vi "FPGA Settings.vi"(8 "error in":errorcluster, 9 "Action":T2, 10 "FPGA Settings":T1={"Bitfile path"=path "", "RIO Device Address"="RIO0", "Group"=FALSE}, 11 "VS Engine in":refnum<class "VS Engine.lvclass">) -> (0 "error out":errorcluster, 2 "FPGA Settings":T1, 3 "VS Engine out":refnum<class "VS Engine.lvclass">)   [LabVIEW 2024, in "VS Engine Abstraction.lvlib" / "VS Engine.lvclass"]
uses:
  VS Engine.lvclass
  VS Engine.lvclass/VS Engine.ctl
  <vilib>/NI VeriStand/Custom Device API/Custom Device API.lvlib
  Addon Shared/SubVIs/Constants.vi
  Addon Shared/FPGA Addon Shared.lvlib
  <vilib>/NI VeriStand/Custom Device API/Set Item Property (Boolean).vi
  <vilib>/NI VeriStand/Custom Device API/Get Item Property (Boolean).vi
  <vilib>/NI VeriStand/Custom Device API/Get Item Property (String).vi
  <vilib>/NI VeriStand/Custom Device API/Set Item Property (String).vi
  <vilib>/NI VeriStand/Custom Device API/Set Item Property (Path).vi
  <vilib>/NI VeriStand/Custom Device API/Get Item Property (Path).vi
  Addon Shared/Types/FPGA Settings.ctl
  Addon Shared/Types/FG Action.ctl
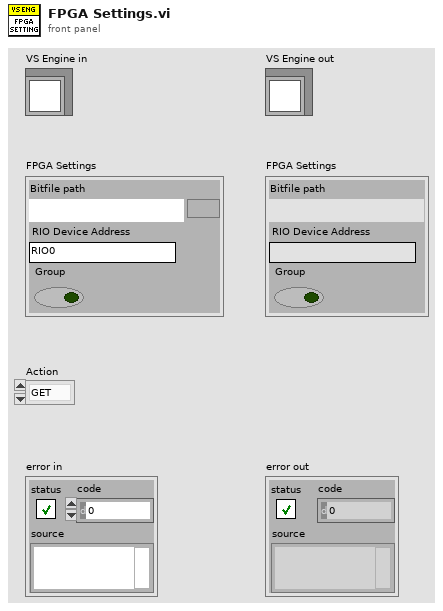
[diagram p1: front panel]
types:
  T1 = typedef "FPGA Addon Shared.lvlib/FPGA Settings.ctl" = cluster{"Bitfile path":path, "RIO Device Address":string, "Group":bool}
  T2 = typedef "FPGA Addon Shared.lvlib/FG Action.ctl" = enum8{"GET", "SET"}
  T3 = typedef "Custom Device API.lvlib/Custom Device Item Ref.ctl" = u64
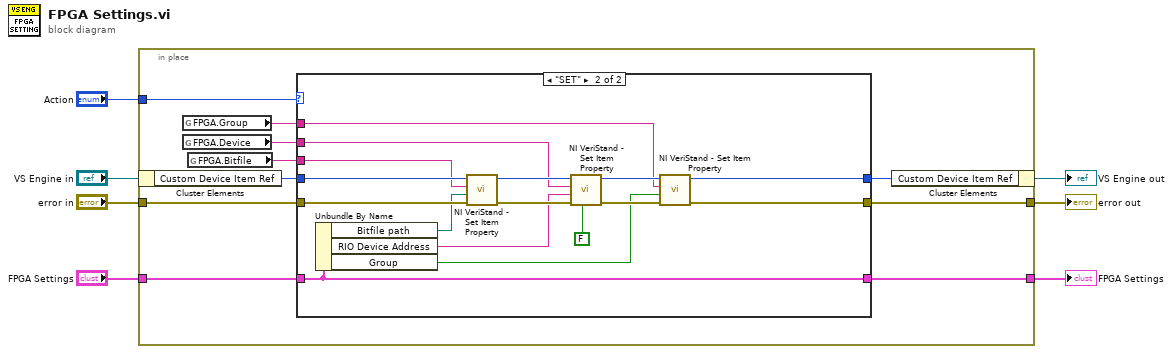
[diagram p0: block diagram]
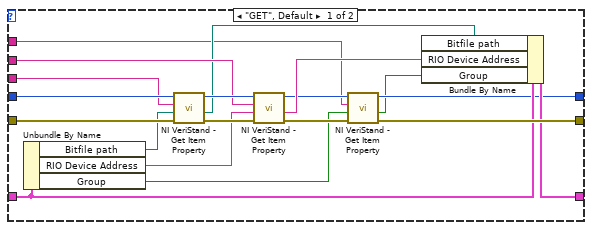
[diagram p2: hidden frame]
diagram:
  n1 = in-place {
    in-place-border: "error in" -> [w17]
    in-place-border: [w16] -> w6
    in-place-border: [w14] -> w5
    in-place-border: "Action" -> [w11]
    in-place-border: "FPGA Settings" -> [w8]
    n2 = in-place-cluster #1("VS Engine in") -> ("Custom Device Item Ref"=w10:T3)
    n3 = global read "Constants.vi" "FPGA.Group"() -> (w12:string)
    n4 = global read "Constants.vi" "FPGA.Device"() -> (w13:string)
    n5 = global read "Constants.vi" "FPGA.Bitfile"() -> (w15:string)
    n6 = case shown="\"SET\"" w11 {
      tunnel: w17 -> [w36 w52]
      tunnel: w10 -> [w32 w48]
      tunnel: w8 -> [w26 w46]
      tunnel: [w33 w49] -> w16
      tunnel: [w21 w39] -> w9
      tunnel: [w25 w46] -> w14
      tunnel: w15 -> [w31 w47]
      tunnel: w13 -> [w27 w41]
      tunnel: w12 -> [w18 w37]
      frame "GET", Default {
        n7 = Unbundle By Name(w26) -> ("Bitfile path"=w29:path, "RIO Device Address"=w28:string, "Group"=w20:bool)
        n8 = call-poly <vilib>:"NI VeriStand - Get Item Property.vi"("error in (no error)"=w36, "Default Value"=w29, "Property Name"=w31, "Item Ref in"=w32) -> ("error out"=w35:errorcluster, "Value"=w24:path, "Item Ref out"=w30:T3)  [unwired: 4 in, 1 out]
        n9 = call-poly <vilib>:"NI VeriStand - Get Item Property.vi"("error in (no error)"=w35, "Default Value"=w28, "Property Name"=w27, "Item Ref in"=w30) -> ("error out"=w34:errorcluster, "Value"=w23:string, "Item Ref out"=w22:T3)  [unwired: 4 in, 1 out]
        n10 = call-poly <vilib>:"NI VeriStand - Get Item Property.vi"("error in (no error)"=w34, "Default Value"=w20, "Property Name"=w18, "Item Ref in"=w22) -> ("error out"=w33:errorcluster, "Value"=w19:bool, "Item Ref out"=w21:T3)  [unwired: 4 in, 1 out]
        n11 = Bundle By Name(cluster=w26, "Bitfile path"=w24, "RIO Device Address"=w23, "Group"=w19) -> (w25:T1)
      }
      frame "SET" {
        n12 = Unbundle By Name(w46) -> ("Bitfile path"=w45:path, "RIO Device Address"=w42:string, "Group"=w38:bool)
        n13 = call-poly <vilib>:"NI VeriStand - Set Item Property.vi"("error in (no error)"=w52, "Value"=w45, "Property Name"=w47, "Item Ref in"=w48) -> ("error out"=w51:errorcluster, "Item Ref out"=w44:T3)  [unwired: 5 in, 1 out]
        n14 = call-poly <vilib>:"NI VeriStand - Set Item Property.vi"("Binary String (T)"=FALSE, "error in (no error)"=w51, "Value"=w42, "Property Name"=w41, "Item Ref in"=w44) -> ("error out"=w50:errorcluster, "Item Ref out"=w40:T3)  [unwired: 4 in, 1 out]
        n15 = call-poly <vilib>:"NI VeriStand - Set Item Property.vi"("error in (no error)"=w50, "Value"=w38, "Property Name"=w37, "Item Ref in"=w40) -> ("error out"=w49:errorcluster, "Item Ref out"=w39:T3)  [unwired: 5 in, 1 out]
      }
    }
    n16 = in-place-cluster #1("Custom Device Item Ref"=w9) -> (→"VS Engine out":refnum<class "VS Engine.lvclass">)
  }
  "error out" <- w6
  "FPGA Settings" <- w5
